vi "create_hypertable.vi"(7 "connection_reference":T2, 8 "error in (no error)":errorcluster, 10 "options":T1={"time_column"="time", "chunk_time_interval"=86400.0} {"chunk_time_interval" format="%<%H:%M:%S>t"}, 11 "table_name":string) -> (0 "error out":errorcluster, 3 "hyper_table_name":string)   [LabVIEW 2015, in "lv-timescaledb.lvlib"]
uses:
  lv-timescaledb.lvlib
  <vilib>/addons/database/Connection.llb/Conn ObjectReference.ctl
  _controls/hypertable_options.ctl
  <vilib>/addons/database/Command.llb/Cmd Execute.vi
  <vilib>/addons/database/Recordset.llb/Rec Fetch Recordset Data (CR).vi
  <vilib>/addons/database/Recordset.llb/Rec Destroy - Command.vi
  <vilib>/addons/database/Command.llb/Cmd Delete.vi
  <vilib>/addons/database/NI_Database_API.lvlib
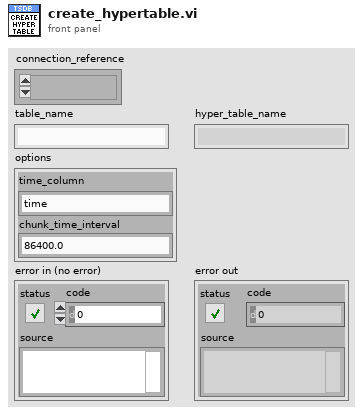
[diagram p1: front panel]
types:
  T1 = typedef "lv-timescaledb.lvlib/hypertable_options.ctl" = cluster{"time_column":string, "chunk_time_interval":dbl}
  T2 = typedef "NI_Database_API.lvlib/Conn ObjectReference.ctl" = refnum<k1>
  T3 = cluster{"table_name":string, "time_column":string}
  T4 = typedef "NI_Database_API.lvlib/DB Tools Parameter Info.ctl" = cluster{"parameter name":string, "type":T5, "direction":T6, "value":variant}
  T5 = typedef "NI_Database_API.lvlib/DB Tools DataTypes.ctl" = enum16{"String", "Long (I32)", "Single (SGL)", "Double (DBL)", "Date/Time", "Binary"}
  T6 = typedef "NI_Database_API.lvlib/DB Tools Parameter Dir.ctl" = enum32{"Input", "Output", "Input/Output", "Return Value"}
  T7 = typedef "NI_Database_API.lvlib/Cmd ObjectReference.ctl" = refnum<k1>
  T8 = typedef "NI_Database_API.lvlib/Cmd-Rec Object Reference.ctl" = refnum<k1>
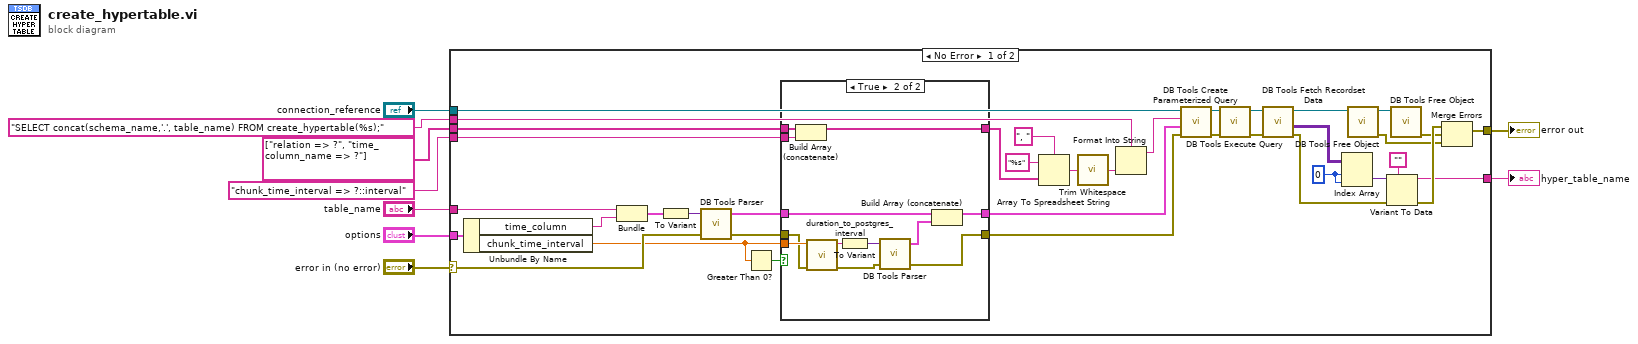
[diagram p0: block diagram]
diagram:
  n1 = case shown="No Error" "error in (no error)" {
    selector: "error in (no error)" -> [w22 w63]
    tunnel: "table_name" -> [w33 _]
    tunnel: "connection_reference" -> [w37 _]
    tunnel: [w47 w63] -> w4
    tunnel: [w28 _] -> w3
    tunnel: "options" -> [w43 _]
    tunnel: "SELECT concat(schema_name,'.', table_name) FROM create_hypertable(%s);" -> [w16 _]
    tunnel: string[] ["relation => ?", "time_column_name => ?"] -> [w18 _]
    tunnel: "chunk_time_interval => ?::interval" -> [w11 _]
    frame No Error {
      w26 = 0 ("disabled index (col)")
      n2 = Unbundle By Name(w43) -> ("time_column"=w32:string, "chunk_time_interval"=w21:dbl)
      n3 = Bundle("table_name"=w33, "time_column"=w32) -> (w31:T3)  [unwired: 1 in]
      n4 = To Variant(anything=w31) -> (Variant=w30:variant)
      n5 = call <vilib>:"DB Tools Parser.vi"("error in (no error)"=w22, "variant"=w30) -> ("error out"=w24:errorcluster, "parameters"=w25:T4[])  [unwired: 2 in]
      n6 = Greater Than 0?(x=w21) -> (x > 0?=w20:bool)
      n7 = case shown="True" w20 {
        tunnel: w25 -> [w50 w56]
        tunnel: w24 -> [w49 w61]
        tunnel: [w49 w54] -> w23
        tunnel: w21 -> [_ w62]
        tunnel: [w50 w55] -> w19
        tunnel: w18 -> [w48 w53]
        tunnel: [w48 w52] -> w17
        tunnel: w11 -> [_ w51]
        frame False {
        }
        frame True {
          n8 = Build Array (concatenate)(w53, w51) -> (w52:string[])
          n9 = call "duration_to_postgres_interval.vi"("error in (no error)"=w61, "relative_time"=w62) -> ("error out"=w58:errorcluster, "interval"=w59:string)  [unwired: 8 in]
          n10 = To Variant(anything=w59) -> (Variant=w60:variant)
          n11 = call <vilib>:"DB Tools Parser.vi"("error in (no error)"=w58, "variant"=w60) -> ("error out"=w54:errorcluster, "parameters"=w57:T4[])  [unwired: 2 in]
          n12 = Build Array (concatenate)(w56, w57) -> (w55:T4[])
        }
      }
      n13 = Array To Spreadsheet String(delimiter (Tab)=", ", array=w17, 3:"%s" ("format string")) -> (spreadsheet string=w14:string)
      n14 = call <vilib>:"Trim Whitespace.vi"("string"=w14) -> ("trimmed string"=w10:string)  [unwired: 1 in]
      n15 = Format Into String(format string=w16, w10) -> (resulting string=w15:string)  [unwired: 2 in, 1 out]
      n16 = call <vilib>:"DB Tools Create Parameterized Query.vi"("error in (no error)"=w23, "parameters"=w19, "SQL query"=w15, "connection reference"=w37) -> ("error out"=w40:errorcluster, "command reference"=w41:T7)  [unwired: 3 in, 1 out]
      n17 = call-poly <vilib>:"DB Tools Execute Query.vi"("error in (no error)"=w40, "command reference"=w41) -> ("error out"=w36:errorcluster, "command-recordset reference"=w38:T8)  [unwired: 6 in]
      n18 = call-poly <vilib>:"DB Tools Fetch Recordset Data.vi"("error in (no error)"=w36, "command-recordset reference"=w38) -> ("error out"=w46:errorcluster, "recordset data"=w44:variant[][], "command-recordset reference out"=w39:T8)  [unwired: 3 in]
      n19 = Index Array(array=w44, index (row)=w26, index (col)=w26) -> (element=w29:variant)
      n20 = call-poly <vilib>:"DB Tools Free Object.vi"("command-recordset reference"=w39) -> ("error out"=w34:errorcluster, "command reference"=w42:T7)  [unwired: 9 in]
      n21 = Variant To Data(error in=w46, type="", Variant=w29) -> (data=w28:string, error out=w45:errorcluster)
      n22 = call-poly <vilib>:"DB Tools Free Object.vi"("command reference"=w42) -> ("error out"=w35:errorcluster)  [unwired: 9 in, 1 out]
      n23 = Merge Errors(w45, w35, w34) -> (w47:errorcluster)
    }
    frame Error {
    }
  }
  "error out" <- w4
  "hyper_table_name" <- w3
